vi "SR530 threshold.vi"(8 "Threshold (mV)":dbl=0.002 min=0.0 max=0.05 step=0.001, 11 "SR530":refnum<visa-resource-name>="COM2") -> (0 "x <= y?":bool, 2 "Abs value (mV)":dbl format="%#.10g")   [LabVIEW 2015]
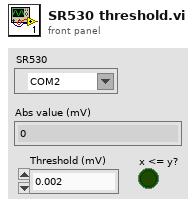
[diagram p1: front panel]
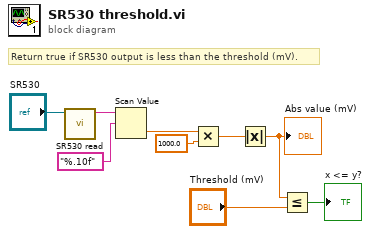
[diagram p0: block diagram]
diagram:
  # "Return true if SR530 output is less than the threshold (mV)."
  n1 = call "SR530 read.vi"("SR530"="SR530") -> ("Result"=w8:string)  [unwired: 10 in]
  n2 = Scan Value(string=w8, format string="%.10f") -> (value=w6:dbl)  [unwired: 1 in, 1 out]
  n3 = Multiply(x=w6, y=1000.0) -> (x*y=w4:dbl)
  n4 = Absolute Value(x=w4) -> (abs(x)=w3:dbl)
  "Abs value (mV)" <- w3
  n5 = Less Or Equal?(x=w3, y="Threshold (mV)") -> (x <= y?=→"x <= y?":bool)
